vi "FTW-Request-Destroy.vi"(0 "FTW-Request In":refnum<class "FTW-Request.lvclass">, 11 "error in":errorcluster) -> (15 "error out":errorcluster)   [LabVIEW 2013, in "FTW-Request.lvclass"]
uses:
  FTW-Request.lvclass
  FTW-Request.lvclass/FTW-Request.ctl
  Endpoint/FTW-Endpoint.lvclass
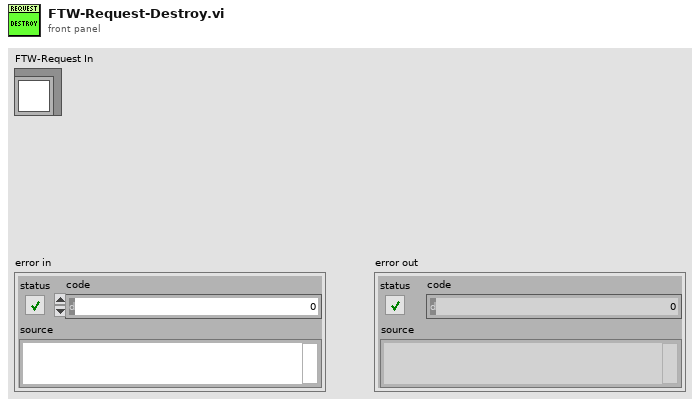
[diagram p1: front panel]
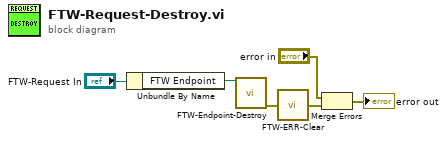
[diagram p0: block diagram]
diagram:
  n1 = Unbundle By Name("FTW-Request In") -> ("FTW Endpoint"=w3:refnum<class "FTW-Endpoint.lvclass">)
  n2 = call-dynamic "FTW-Endpoint-Destroy.vi"("FTW Endpoint"=w3) -> ("error out"=w2:errorcluster)  [unwired: 14 in]
  n3 = call "FTW-ERR-Clear.vi"("error to snuff"=w2) -> ("no error"=w1:errorcluster)
  n4 = Merge Errors("error in", w1) -> (→"error out":errorcluster)
